vi "Configure.vi"(8 "error in (no error)":errorcluster, 11 "Strain in":refnum<class "Strain.lvclass">) -> (0 "error out":errorcluster, 3 "Strain out":refnum<class "Strain.lvclass">)   [LabVIEW 2015, in "Strain.lvlib" / "Strain.lvclass"]
uses:
  Strain.lvclass
  <userlib>/Common Components/Measurement Actor/Measurement.lvclass/Measurement.ctl
  <userlib>/Common Components/Measurement Actor/Measurement.lvclass
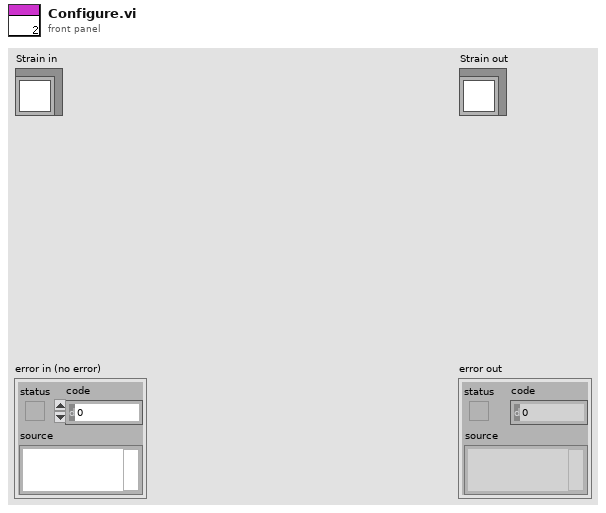
[diagram p1: front panel]
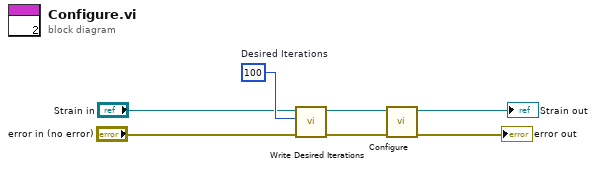
[diagram p0: block diagram]
diagram:
  w5 = 100  # Desired Iterations
  n1 = call <userlib>:"Write Desired Iterations.vi"("error in (no error)"="error in (no error)", "Desired Iterations"=w5, "Measurement in"="Strain in") -> ("error out"=w4:errorcluster, "Measurement out"=w6:refnum<class "Strain.lvclass">)  [unwired: 7 in]
  n2 = call-parent "Configure.vi"("error in (no error)"=w4, "Measurement in"=w6) -> ("error out"=→"error out":errorcluster, "Measurement out"=→"Strain out":refnum<class "Strain.lvclass">)  [unwired: 8 in]
